vi "main.vi"() -> ()   [LabVIEW 2023]
panel:
  out "?":u16[](graph)
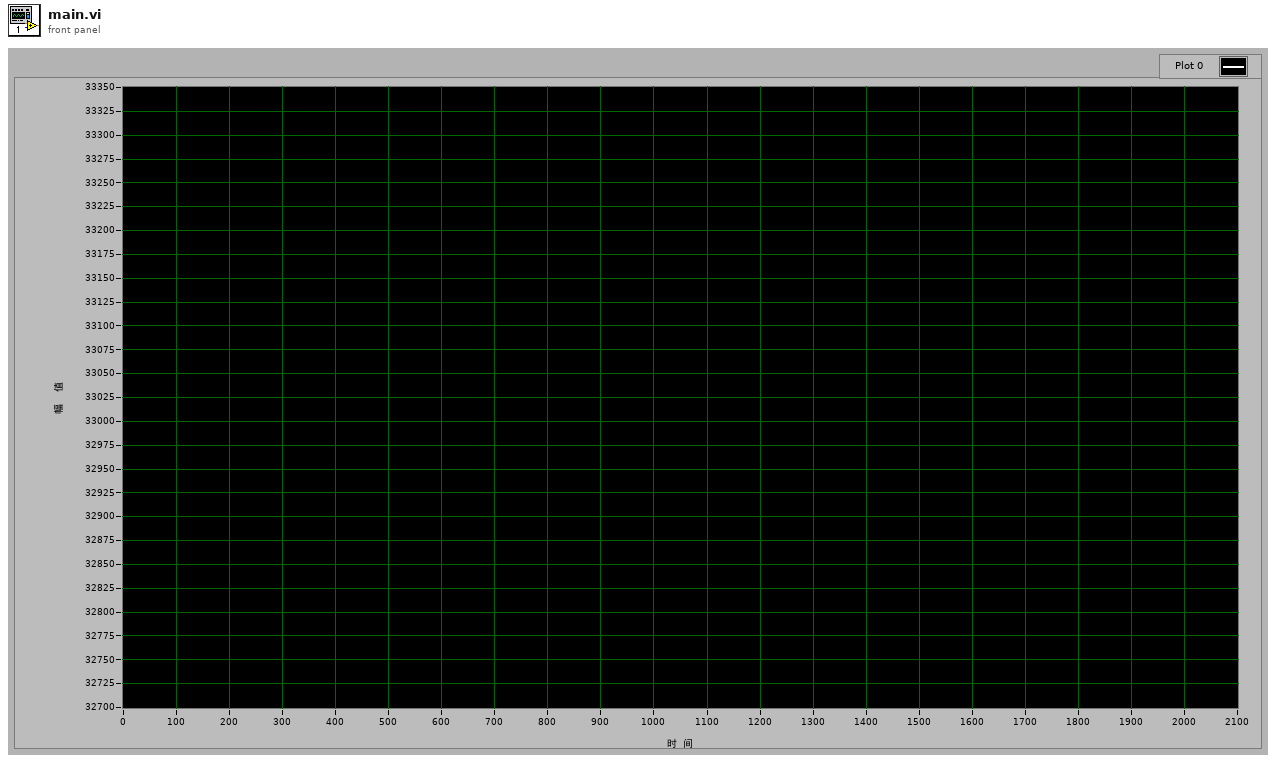
[diagram p1: front panel]
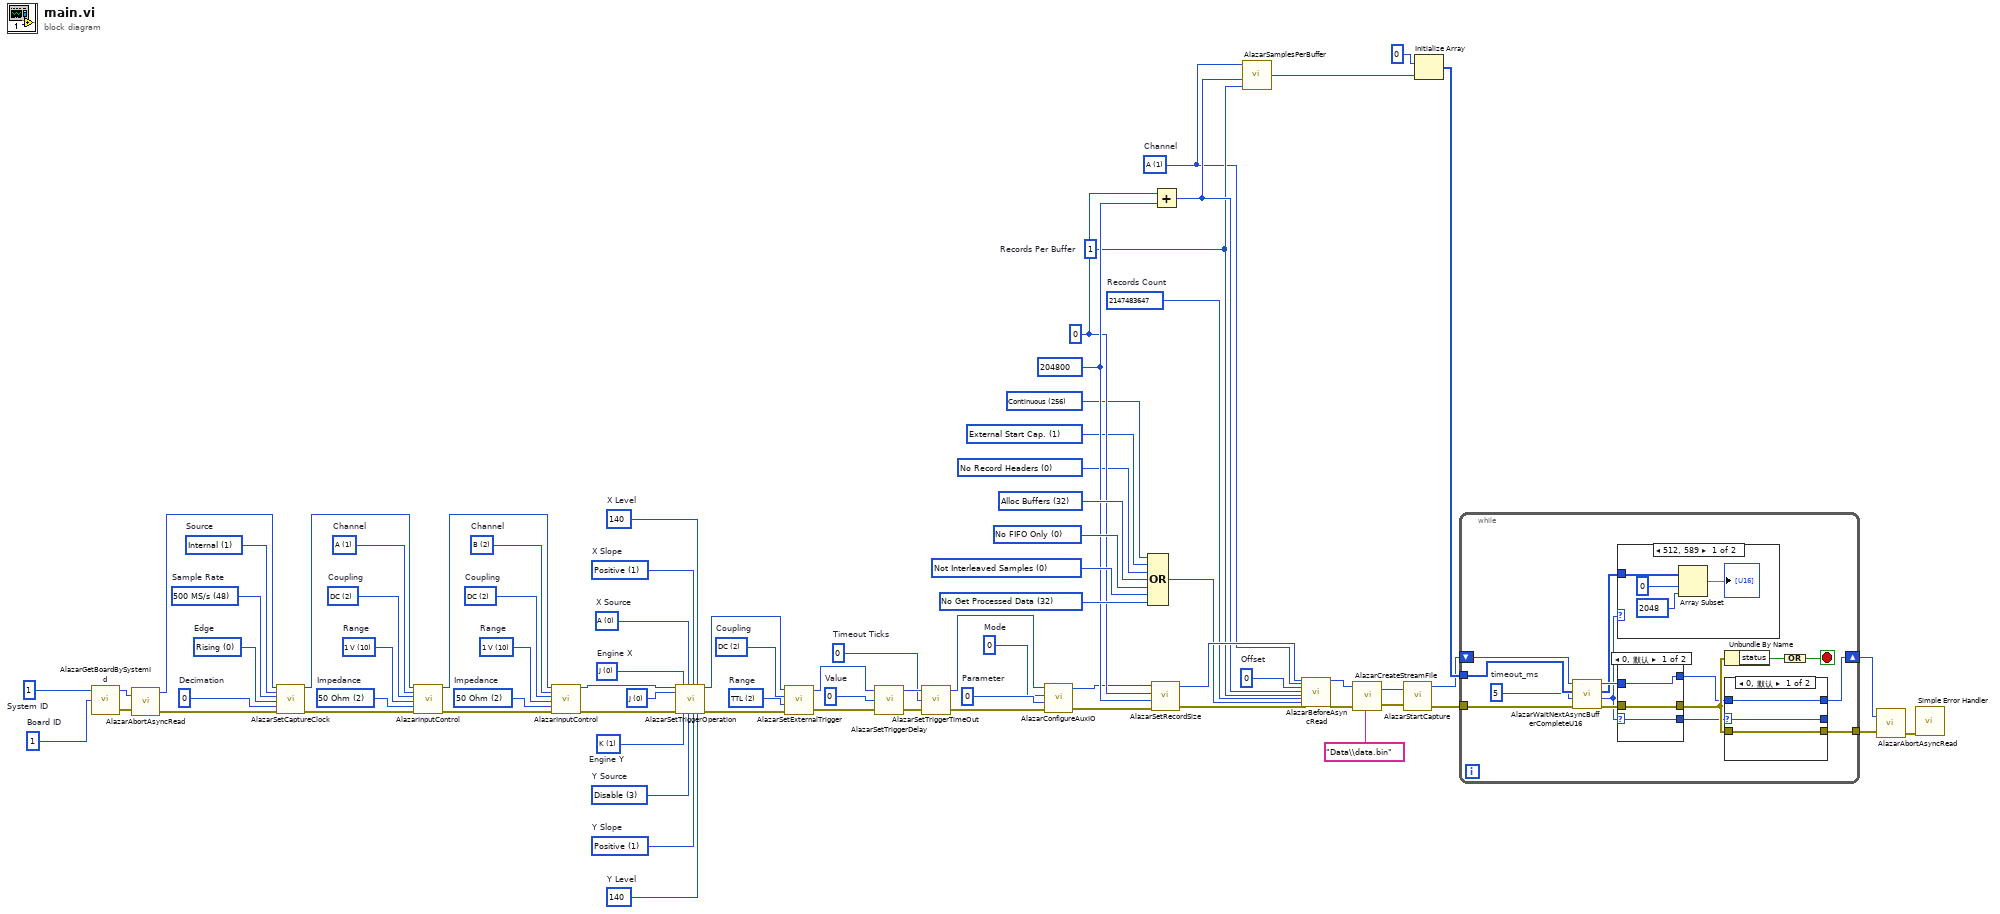
[diagram p0: block diagram]
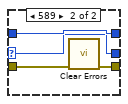
[diagram p3: hidden frame]
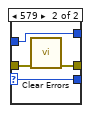
[diagram p4: hidden frame]
diagram:
  w31 = u32 2 items=["50 Ohm"=2]  # Impedance
  w30 = u32 10 items=["40 mV"=2, "100 mV"=5, "200 mV"=6, "400 mV"=7, "1 V"=10, "2 V"=11, "4 V"=12]  # Range
  w32 = u32 2 items=["AC"=1, "DC"=2]  # Coupling
  w33 = u8 2 items=["A"=1, "B"=2, "C"=4, "D"=8]  # Channel
  w9 = u32 0  # Parameter
  w8 = u32 0  # Mode
  w7 = u32 0  # Timeout Ticks
  w14 = u32 0  # Value
  w18 = u32 2 items=["5 V"=0, "TTL"=2, "2.5V, 50Ohm"=3]  # Range
  w17 = u32 2 items=["AC"=1, "DC"=2]  # Coupling
  w21 = u32 140  # Y Level
  w22 = u32 1 items=["Positive"=1, "Negative"=2]  # Y Slope
  w23 = u32 3 items=["A", "B", "External", "Disable", "C", "D"]  # Y Source
  w25 = u32 140  # X Level
  w26 = u32 1 items=["Positive"=1, "Negative"=2]  # X Slope
  w27 = u32 0 items=["A", "B", "External", "Disable", "C", "D"]  # X Source
  w24 = u32 1 items=["J", "K"]  # Engine Y
  w28 = u32 0 items=["J", "K"]  # Engine X
  w29 = u32 0 items=["J", "K", "J OR K", "J AND K", "J XOR K", "J AND NOT K", "NOT J AND K"] ("Op.")
  w36 = u32 2 items=["50 Ohm"=2]  # Impedance
  w37 = u32 10 items=["40 mV"=2, "100 mV"=5, "200 mV"=6, "400 mV"=7, "1 V"=10, "2 V"=11, "4 V"=12]  # Range
  w38 = u32 2 items=["AC"=1, "DC"=2]  # Coupling
  w39 = u8 1 items=["A"=1, "B"=2, "C"=4, "D"=8]  # Channel
  w41 = u32 0  # Decimation
  w42 = u32 0 items=["Rising", "Falling"]  # Edge
  w43 = u32 48 items=["1 kS/s"=1, "2 kS/s"=2, "5 kS/s"=4, "10 kS/s"=8, "20 kS/s"=10, "50 kS/s"=12, "100 kS/s"=14, "200 kS/s"=16, "500 kS/s"=18, "1 MS/s"=20, "2 MS/s"=24, "5 MS/s"=26, "10 MS/s"=28, "20 MS/s"=30, "50 MS/s"=34, "100 MS/s"=36, "125 MS/s"=37, "250 MS/s"=43, "500 MS/s"=48, "USER_DEF"=0]  # Sample Rate
  w45 = u32 1 items=["Internal"=1, "Fast External"=2, "Medium External"=3, "Slow External"=4, "External AC"=5, "External DC"=6, "External 10MHz"=7]  # Source
  w49 = u32 1  # Board ID
  w48 = u32 1  # System ID
  w57 = u32 1 items=["A"=1, "B"=2, "A, B"=3]  # Channel
  w64 = u32 0 items=["No Record Headers"=0, "Enable Record Headers"=8]
  w61 = u32 2147483647  # Records Count
  w58 = u32 1  # Records Per Buffer
  w70 = u32 0  # Offset
  w75 = u32 204800 ("Post-trigger Samples")
  w74 = u32 0 ("Pre-trigger Samples")
  w79 = u32 32 items=["No Get Processed Data"=32, "Get Processed Data"=8192]
  w78 = u32 0 items=["Not Interleaved Samples"=0, "Interleave Samples"=4096]
  w76 = u32 0 items=["No FIFO Only"=0, "FIFO Only"=2048]
  w77 = u32 32 items=["Alloc Buffers"=32]
  w63 = u32 1 items=["Internal Start Cap.", "External Start Cap."]
  w62 = u32 256 items=["Traditional"=0, "NPT"=512, "Continuous"=256, "Triggered Streaming"=1024]
  n1 = call "AlazarGetBoardBySystemId.vi"("Board ID"=w49, "System ID"=w48) -> ("error out"=w46:errorcluster, "Handle"=w47:u64)  [unwired: 1 in, 1 out]
  n2 = call "AlazarAbortAsyncRead.vi"("Handle"=w47, "error in (no error)"=w46) -> ("Handle"=w44:u64, "error out"=w40:errorcluster)  [unwired: 1 out]
  n3 = call "AlazarSetCaptureClock.vi"("Handle"=w44, "Source"=w45, "Sample Rate"=w43, "Edge"=w42, "Decimation"=w41, "error in (no error)"=w40) -> ("Handle"=w35:u64, "error out"=w34:errorcluster)  [unwired: 11 in, 1 out]
  n4 = call "AlazarInputControl.vi"("Handle"=w35, "Channel"=w39, "Coupling"=w38, "Range"=w37, "Impedance"=w36, "error in (no error)"=w34) -> ("Handle"=w6:u64, "error out"=w5:errorcluster)  [unwired: 11 in, 1 out]
  n5 = call "AlazarInputControl.vi"("Handle"=w6, "Channel"=w33, "Coupling"=w32, "Range"=w30, "Impedance"=w31, "error in (no error)"=w5) -> ("Handle"=w3:u64, "error out"=w4:errorcluster)  [unwired: 11 in, 1 out]
  n6 = call "AlazarSetTriggerOperation.vi"("Handle"=w3, "Trigger Operation"=w29, "error in (no error)"=w4, "Trigger Engine 1"=w28, "Trigger Engine 2"=w24, "Source 1"=w27, "Source 2"=w23, "Slope 1"=w26, "Slope 2"=w22, "Level 1"=w25, "Level 2"=w21) -> ("Handle"=w20:u64, "error out"=w19:errorcluster)  [unwired: 6 in, 1 out]
  n7 = call "AlazarSetExternalTrigger.vi"("error in (no error)"=w19, "Range ID"=w18, "Coupling ID"=w17, "Handle"=w20) -> ("error out"=w15:errorcluster, "Handle"=w16:u64)  [unwired: 1 out]
  n8 = call "AlazarSetTriggerDelay.vi"("error in (no error)"=w15, "Delay"=w14, "Handle"=w16) -> ("error out"=w12:errorcluster, "Handle"=w13:u64)  [unwired: 1 out]
  n9 = call "AlazarSetTriggerTimeOut.vi"("error in (no error)"=w12, "Timeout Ticks"=w7, "Handle"=w13) -> ("error out"=w10:errorcluster, "Handle"=w11:u64)  [unwired: 1 out]
  n10 = call "AlazarConfigureAuxIO.vi"("error in (no error)"=w10, "Parameter"=w9, "Mode"=w8, "Handle"=w11) -> ("error out"=w2:errorcluster, "Handle"=w1:u64)  [unwired: 1 out]
  n11 = Compound Arithmetic op=OR(w62, w63, w64, w77, w76, w78, w79) -> (w71:u32)
  n12 = call "AlazarSetRecordSize.vi"("error in (no error)"=w2, "Post-trigger Samples"=w75, "Pre-trigger Samples"=w74, "Handle"=w1) -> ("error out"=w72:errorcluster, "Handle"=w73:u64)  [unwired: 1 out]
  n13 = Add(x=w74, y=w75) -> (x+y=w59:u32)
  n14 = call "AlazarSamplesPerBuffer.vi"("Records Per Buffer"=w58, "Samples Per Record"=w59, "Channel Mask"=w57) -> ("Samples Per Buffer"=w60:u32)  [unwired: 1 in]
  n15 = call "AlazarBeforeAsyncRead.vi"("Handle"=w73, "Channel Select"=w57, "Transfer Offset"=w70, "Transfer Length"=w59, "Records Per Buffer"=w58, "Records Per Acquisition"=w61, "Flags"=w71, "error in (no error)"=w72) -> ("Handle"=w53:u64, "error out"=w51:errorcluster)  [unwired: 17 in, 1 out]
  n16 = call "AlazarCreateStreamFile.vi"("error in (no error)"=w51, "File Path"="Data\\data.bin", "Handle"=w53) -> ("error out"=w55:errorcluster, "Handle"=w56:u64)
  n17 = call "AlazarStartCapture.vi"("Handle"=w56, "error in (no error)"=w55) -> ("Handle"=w52:u64, "error out"=w50:errorcluster)  [unwired: 1 out]
  n18 = Initialize Array(u16 0, w60) -> (w68:u16[])
  n19 = while {
    tunnel: w68 -> [w94]
    tunnel: w50 -> [w91]
    tunnel: [w86] -> w65
    shift-right: [w87] -> w66
    shift-left: w52 -> [w93]
    stop <- w84 stop-if-true
    w92 = u32 5  # timeout_ms
    n20 = call "AlazarWaitNextAsyncBufferCompleteU16.vi"("error in (no error)"=w91, "Timeout (ms)"=w92, "Buffer"=w94, "Handle"=w93) -> ("error out"=w83:errorcluster, "Return Code"=w80:u32, "Buffer"=w81:u16[], "Handle"=w82:u64)
    n21 = case shown="512, 589" w80 {
      tunnel: w81 -> [w95 _]
      frame 512, 589 {
        n22 = Array Subset(array=w95, index=0, length=2048) -> (→"?":u16[])
      }
      frame Default {
      }
    }
    n23 = case shown="0, 默认" w80 {
      selector: w80 -> [w107 w109]
      tunnel: w83 -> [w106 w112]
      tunnel: [w106 w111] -> w90
      tunnel: [w108 w110] -> w89
      tunnel: w82 -> [w108 w110]
      tunnel: [w107 w109] -> w88
      frame 0, Default {
      }
      frame 579 {
        n24 = call <vilib>:"Clear Errors.vi"("error in (no error)"=w112) -> ("error out"=w111:errorcluster)  [unwired: 5 in, 1 out]
      }
    }
    n25 = Unbundle By Name(w90) -> ("status"=w85:bool)
    n26 = case shown="0, 默认" w88 {
      selector: w88 -> [w100 w102]
      tunnel: w90 -> [w99 w105]
      tunnel: [w99 w104] -> w86
      tunnel: [w101 w103] -> w87
      tunnel: w89 -> [w101 w103]
      tunnel: [w100 w102] -> _
      frame 0, Default {
      }
      frame 589 {
        n27 = call <vilib>:"Clear Errors.vi"("error in (no error)"=w105) -> ("error out"=w104:errorcluster)  [unwired: 5 in, 1 out]
      }
    }
    n28 = Compound Arithmetic op=OR(w85) -> (w84:bool)
  }
  n29 = call "AlazarAbortAsyncRead.vi"("Handle"=w66, "error in (no error)"=w65) -> ("error out"=w67:errorcluster)  [unwired: 2 out]
  n30 = call <vilib>:"Simple Error Handler.vi"("error in (no error)"=w67) -> ()  [unwired: 4 in, 5 out]
